vi "STOPheat.vi"(0 "connection ID":refnum<k5>, 1 "SEQ in":u32, 2 "error in (no error)":errorcluster) -> (3 "connection ID out":refnum<k5>, 4 "SEQ out":u32, 5 "OK?":bool, 6 "error out":errorcluster)   [LabVIEW 2016]
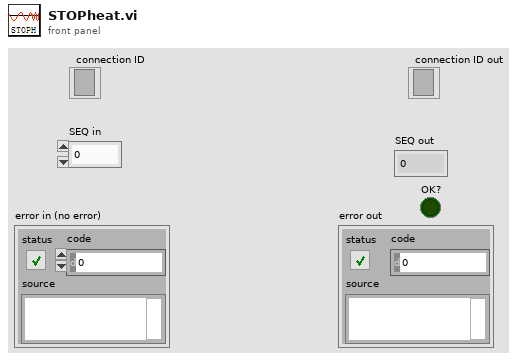
[diagram p1: front panel]
types:
  T1 = enum8{"SET_FREQ", "SET_VOLT", "SET_CHANNEL_VOLT", "SET_PHASE", "START_HEAT", "STOP_HEAT", "CHANNEL_CTRL_SINGLE", "CHANNEL_CTRL_ALL", "READ_VOLT_SET", "READ_VOLT_SET_RSP", "READ_CURRENT_VOLT", "READ_CURRENT_VOLT_RSP", "READ_PHASE", "READ_PHASE_RSP", "READ_HEATTIME_LEFT", "READ_HEATTIME_LEFT_RSP", "EXEC_RSP"}
  T2 = enum8{"SET_FREQ", "SET_VOLT", "SET_CHENNEL_VOLT", "SET_PHASE", "START_HEAT", "STOP_HEAT", "CHANNEL_CTRL_SINGLE", "CHANNEL_CTRL_ALL", "READ_VOLT_SET", "READ_VOLT_SET_RSP", "READ_CURRENT_VOLT", "READ_CURRENT_VOLT_RSP", "READ_PHASE", "READ_PHASE_RSP", "READ_HEATTIME_LEFT", "READ_HEATTIME_LEFT_RSP", "EXEC_RSP"}
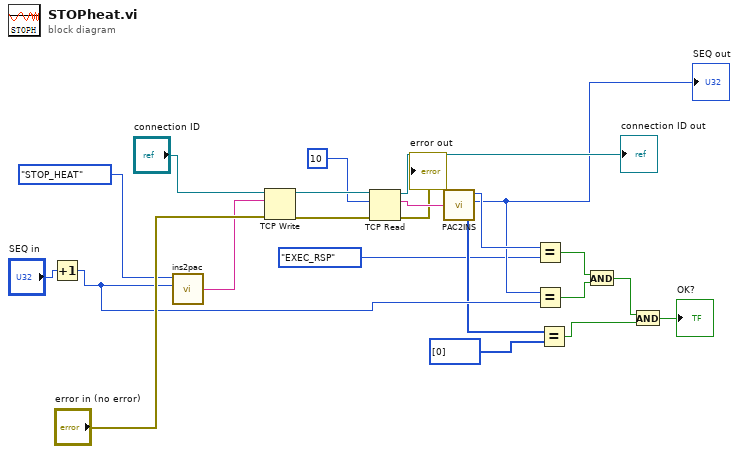
[diagram p0: block diagram]
diagram:
  n1 = Increment(x="SEQ in") -> (x+1=w11:u32)
  n2 = call "ins2pac.vi"("SEQUENCE"=w11, "TYPE"=T1."STOP_HEAT") -> ("PACKET"=w20:string)  [unwired: 2 in]
  n3 = TCP Write(connection ID="connection ID", data in=w20, error in (no error)="error in (no error)") -> (connection ID out=w19:refnum<k5>, error out=w17:errorcluster)  [unwired: 1 in, 1 out]
  n4 = TCP Read(connection ID=w19, bytes to read=10, error in (no error)=w17) -> (connection ID out=→"connection ID out":refnum<k5>, data out=w16:string, error out=→"error out":errorcluster)  [unwired: 2 in]
  n5 = call "PAC2INS.vi"("PACKET"=w16) -> ("TYPE"=w14:T2, "SEQUENCE"=w13:u32, "BODY"=w10:u8[])  [unwired: 1 out]
  "SEQ out" <- w13
  n6 = Equal?(x=w14, y=T1."EXEC_RSP" ("TYPE")) -> (x = y?=w8:bool)
  n7 = Equal?(x=w13, y=w11) -> (x = y?=w7:bool)
  n8 = Equal?(x=w10, y=u8[] [0]) -> (x = y?=w6:bool)
  n9 = And(x=w8, y=w7) -> (x .and. y?=w5:bool)
  n10 = And(x=w5, y=w6) -> (x .and. y?=→"OK?":bool)
